vi "DataWks.vi"(0 "Origin.IOApplication":refnum<k7>, 1 "2d Data":sgl[][](array[numeric]) format="%0.3f", 2 "error in (no error)":errorcluster) -> (3 "Origin.IOApplication":refnum<k7>, 4 "Input Data":cluster{"data":dbl[], "data":dbl[]}(graph), 5 "DataWks":refnum<k7>, 6 "error out":errorcluster)   [LabVIEW 2014]
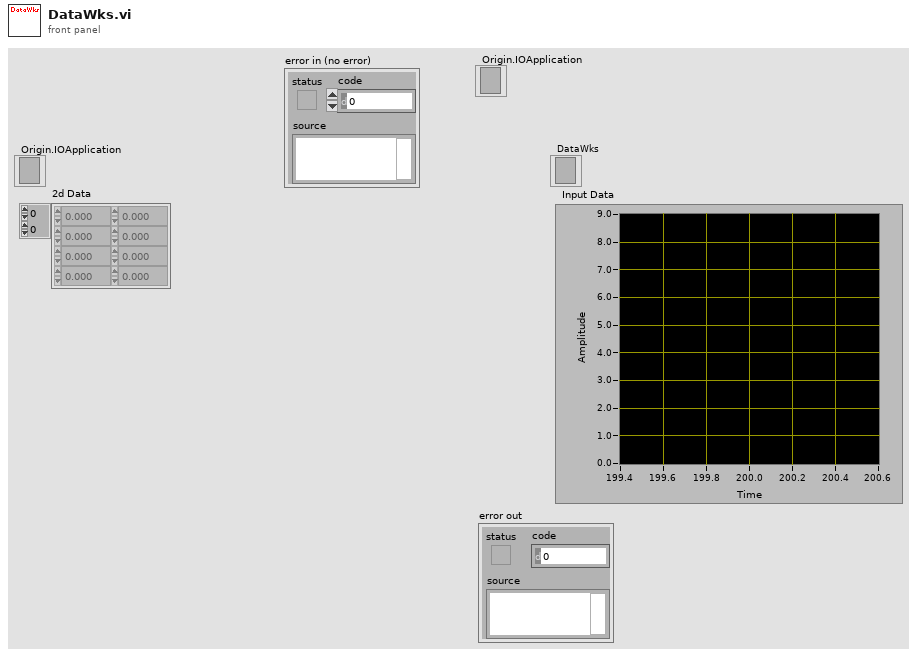
[diagram p1: front panel]
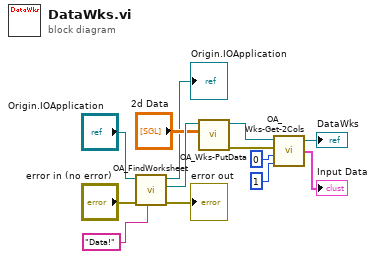
[diagram p0: block diagram]
diagram:
  n1 = call <vilib>:"OA_FindWorksheet.vi"("Name"="Data!", "error in (no error)"="error in (no error)", "Origin.IOApplication"="Origin.IOApplication") -> ("error out"=→"error out":errorcluster, "Origin.Worksheet"=w12:refnum<k7>, "Origin.IOApplication"=→"Origin.IOApplication":refnum<k7>)  [unwired: 6 in]
  n2 = call <vilib>:"OA_Wks-PutData.vi"("2d Data"="2d Data", "Origin.Worksheet"=w12) -> ("error out"=w5:errorcluster, "Origin.Worksheet Out"=w6:refnum<k7>)  [unwired: 3 in, 1 out]
  n3 = call <vilib>:"OA_Wks-Get-2Cols.vi"("yCol"=1, "xCol"=0, "error in (no error)"=w5, "Origin.Worksheet"=w6) -> ("Bundled Cols"=→"Input Data":cluster{"data":dbl[], "data":dbl[]}, "Origin.Worksheet Dup"=→"DataWks":refnum<k7>)  [unwired: 1 out]
